vi "Terminal-PressureSystem-SelfCheck.vi"(8 "error in (no error)":errorcluster caption="错误输入（无错误）") -> (0 "error out":errorcluster caption="错误输出")   [LabVIEW 2014]
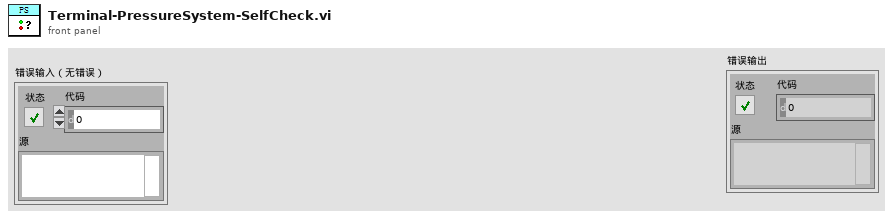
[diagram p1: front panel]
types:
  T1 = cluster{"径向液压缸加载力":u16, "轴向液压缸加载力":u16, "报警信息":cluster{"比例加载油箱液位高":bool, "比例加载油箱液位低":bool, "比例加载高压滤油发讯":bool, "比例加载回油滤油发讯":bool, "比例加载油箱温度发讯":bool}}
  T2 = cluster{"比例加载油箱液位高":bool, "比例加载油箱液位低":bool, "比例加载高压滤油发讯":bool, "比例加载回油滤油发讯":bool, "比例加载油箱温度发讯":bool}
  T3 = cluster{"供油压力":u16, "供油流量":u16, "供油温度":u16, "报警信息":cluster{"主油箱液位高":bool, "主油箱液位低":bool, "副油箱液位高":bool, "副油箱液位低":bool, "回油滤油发讯":bool, "管路滤油发讯":bool, "回油滤油发讯":bool, "吸油滤油发讯":bool, "主油箱温度发讯":bool, "副油箱温度发讯":bool}}
  T4 = cluster{"主油箱液位高":bool, "主油箱液位低":bool, "副油箱液位高":bool, "副油箱液位低":bool, "回油滤油发讯":bool, "管路滤油发讯":bool, "回油滤油发讯":bool, "吸油滤油发讯":bool, "主油箱温度发讯":bool, "副油箱温度发讯":bool}
  T5 = cluster{"高压供油压力":u16, "高压供油流量":u16, "高压供油温度":u16, "低压供油压力":u16, "低压供油流量":u16, "低压供油温度":u16, "报警信息":cluster{"油箱液位高":bool, "油箱液位低":bool, "管路滤油发讯":bool, "回油滤油发讯":bool, "回油滤油发讯":bool, "吸油滤油发讯":bool, "油箱温度发讯":bool}}
  T6 = cluster{"油箱液位高":bool, "油箱液位低":bool, "管路滤油发讯":bool, "回油滤油发讯":bool, "回油滤油发讯":bool, "吸油滤油发讯":bool, "油箱温度发讯":bool}
  T7 = cluster{"加热装置异常报警":bool, "陪试润滑-MA1电机过热":bool, "陪试润滑-MA2电机过热":bool, "陪试润滑-MA3电机过热":bool, "试验润滑-MA1电机过热":bool, "试验润滑-MA2电机过热":bool, "试验润滑-MA3电机过热":bool, "试验润滑-MA4电机过热":bool, "试验润滑-MA5电机过热":bool, "试验润滑-MA6电机过热":bool, "比例加载-MA1电机过热":bool, "比例加载-MA2电机过热":bool}
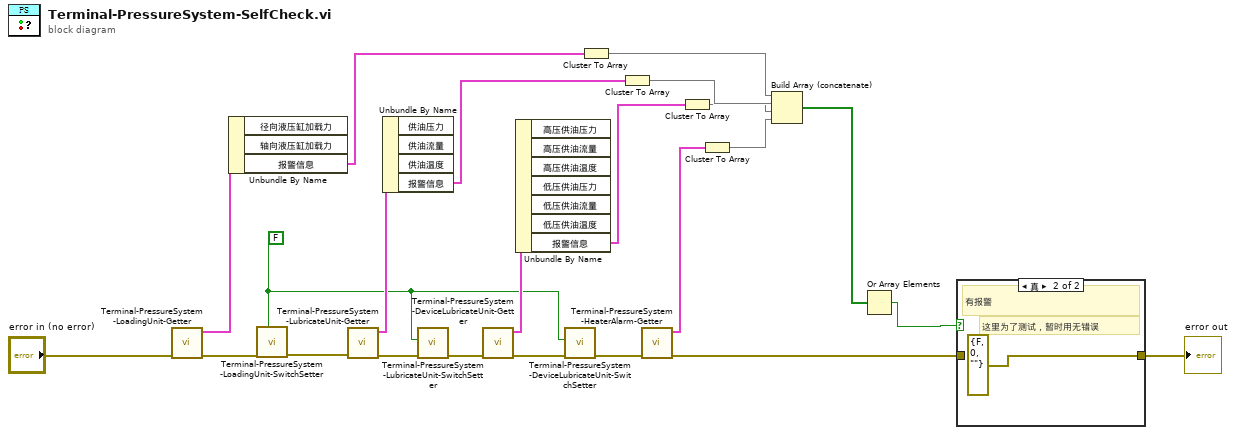
[diagram p0: block diagram]
diagram:
  w13 = FALSE ("启停")
  n1 = call "Terminal-PressureSystem-LoadingUnit-Getter.vi"("error in (no error)"="error in (no error)") -> ("error out"=w19:errorcluster, "液压子系统比例加载单元"=w22:T1)  [unwired: 8 in, 1 out]
  n2 = Unbundle By Name(w22) -> ("报警信息"=w11:T2)  [unwired: 2 out]
  n3 = call "Terminal-PressureSystem-LoadingUnit-SwitchSetter.vi"("error in (no error)"=w19, "启停"=w13) -> ("error out"=w18:errorcluster)  [unwired: 9 in]
  n4 = call "Terminal-PressureSystem-LubricateUnit-Getter.vi"("error in (no error)"=w18) -> ("error out"=w17:errorcluster, "液压子系统试验轴承润滑单元"=w21:T3)  [unwired: 8 in, 1 out]
  n5 = Unbundle By Name(w21) -> ("报警信息"=w10:T4)  [unwired: 3 out]
  n6 = call "Terminal-PressureSystem-LubricateUnit-SwitchSetter.vi"("error in (no error)"=w17, "启停"=w13) -> ("error out"=w16:errorcluster)  [unwired: 9 in]
  n7 = call "Terminal-PressureSystem-DeviceLubricateUnit-Getter.vi"("error in (no error)"=w16) -> ("error out"=w15:errorcluster, "液压子系统陪试润滑单元"=w20:T5)  [unwired: 8 in, 1 out]
  n8 = Unbundle By Name(w20) -> ("报警信息"=w9:T6)  [unwired: 6 out]
  n9 = call "Terminal-PressureSystem-DeviceLubricateUnit-SwitchSetter.vi"("error in (no error)"=w15, "启停"=w13) -> ("error out"=w14:errorcluster)  [unwired: 9 in]
  n10 = Cluster To Array(cluster=w11) -> (array=w8:bool[])
  n11 = Cluster To Array(cluster=w10) -> (array=w7:bool[])
  n12 = call "Terminal-PressureSystem-HeaterAlarm-Getter.vi"("error in (no error)"=w14) -> ("error out"=w1:errorcluster, "加热装置异常信息"=w12:T7)  [unwired: 8 in, 1 out]
  n13 = Cluster To Array(cluster=w9) -> (array=w6:bool[])
  n14 = Cluster To Array(cluster=w12) -> (array=w5:bool[])
  n15 = Build Array (concatenate)(w8, w7, w6, w5) -> (w4:bool[])
  n16 = Or Array Elements(Boolean array=w4) -> (logical OR=w2:bool)
  n17 = case shown="真" w2 {
    tunnel: [w24 errorcluster {"status"=FALSE, "code"=0, "source"=""} ("错误常量")] -> w3
    tunnel: w1 -> [w24 _]
    frame False {
      # "没有报警"
    }
    frame True {
      # "这里为了测试，暂时用无错误"
      # "有报警"
    }
  }
  "error out" <- w3
